vi "SetHead.vi"(0 "object in":refnum<class "Snake.lvclass">, 1 "Head":T1, 5 "error in (no error)":errorcluster) -> (14 "object out":refnum<class "Snake.lvclass">, 19 "error out":errorcluster)   [LabVIEW 2021, in "Snake.lvclass"]
uses:
  Snake.lvclass
  Coordinates.ctl
  Snake.lvclass/Snake.ctl
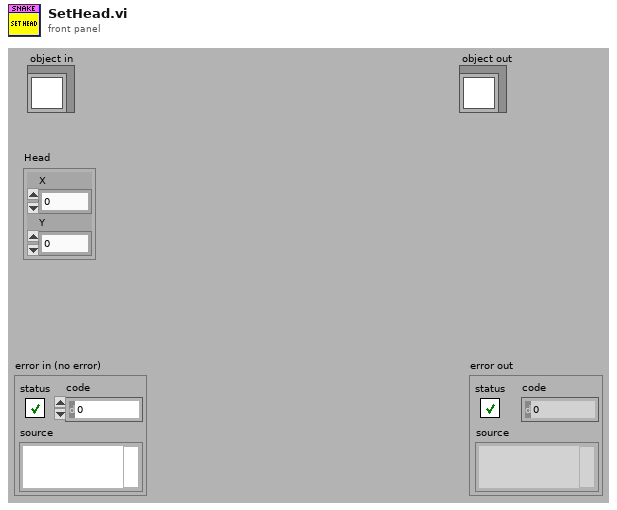
[diagram p1: front panel]
types:
  T1 = typedef "Coordinates.ctl" = cluster{"X":i32, "Y":i32}
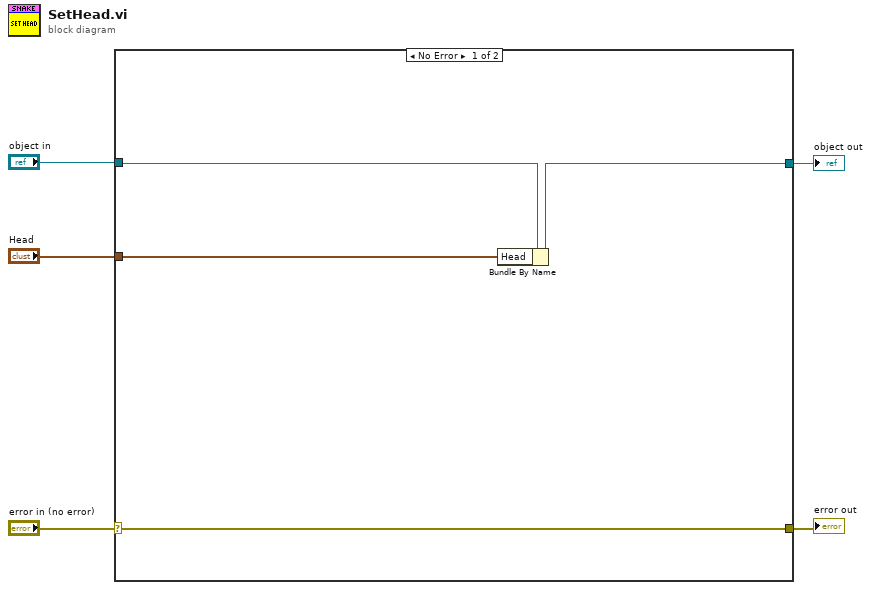
[diagram p0: block diagram]
diagram:
  n1 = case shown="No Error" "error in (no error)" {
    selector: "error in (no error)" -> [w8 w11]
    tunnel: [w8 w11] -> w4
    tunnel: [w6 w10] -> w2
    tunnel: "object in" -> [w7 w10]
    tunnel: "Head" -> [w9 _]
    frame No Error {
      n2 = Bundle By Name(cluster=w7, "Head"=w9) -> (w6:refnum<class "Snake.lvclass">)
    }
    frame Error {
    }
  }
  "error out" <- w4
  "object out" <- w2
